vi "Kelvinox_Set_T_Setpoint.vi"(8 "error in (no error)":errorcluster, 10 "Kelvinox-Cluster":T2, 11 "Connection Details (in)":T1={"Mode"=enum."Immediate", "Bytes to Read"=5000, "IP Address"="172.25.187.107", "Remote Port"=33576, "Timeout"=10000, "connection ID"=refnum}) -> (0 "error out":errorcluster)   [LabVIEW 2019]
uses:
  Monitor Communication/Kelvinox/Kelvinox_Control.ctl
  Instrument_Setup.vi
panel:
  # "Pressures in mbar"
  # "Temperatures in K"
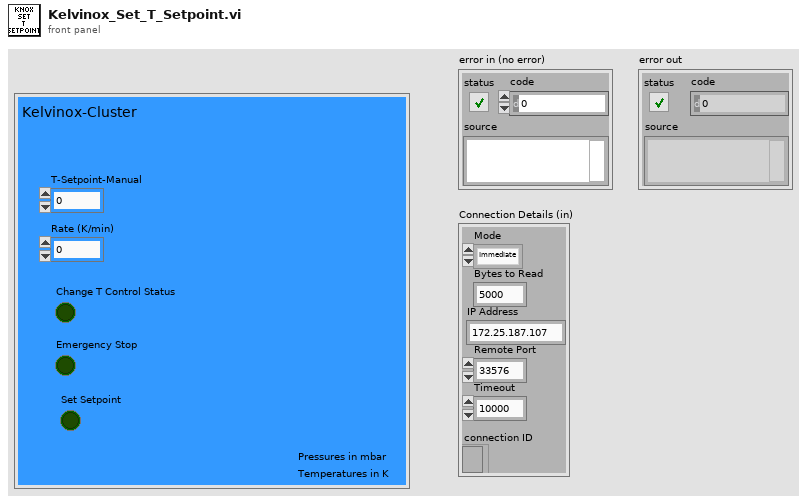
[diagram p1: front panel]
types:
  T1 = cluster{"Mode":enum16{"Standard", "Buffered", "CRLF", "Immediate"}, "Bytes to Read":i32, "IP Address":string, "Remote Port":i32, "Timeout":i32, "connection ID":refnum<k5>}
  T2 = typedef "Kelvinox_Control.ctl" = cluster{"T-Setpoint-Manual":dbl, "Rate (K/min)":dbl, "Change T Control Status":bool, "Emergency Stop":bool, "Set Setpoint":bool}
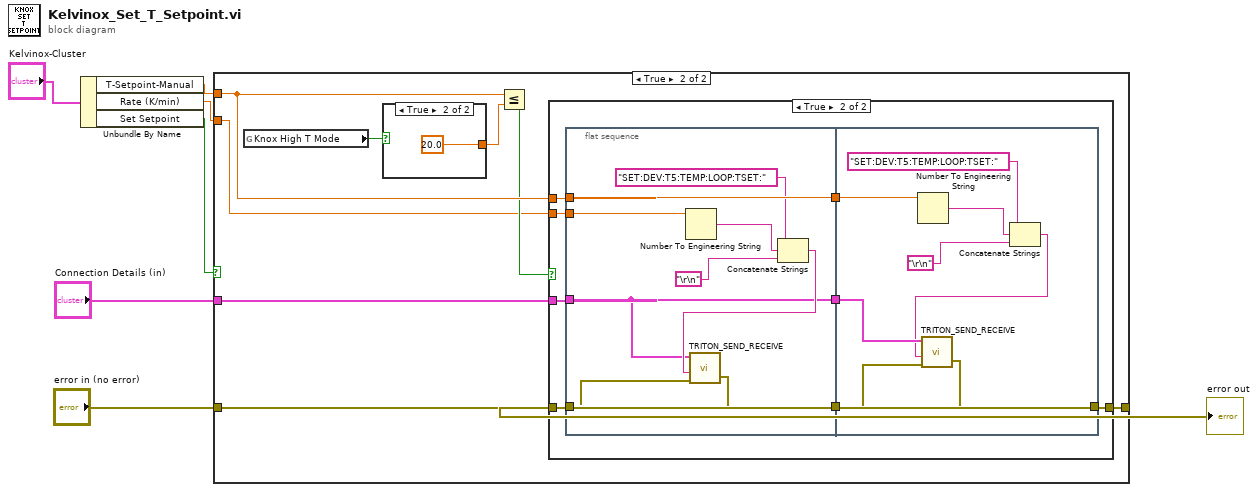
[diagram p0: block diagram]
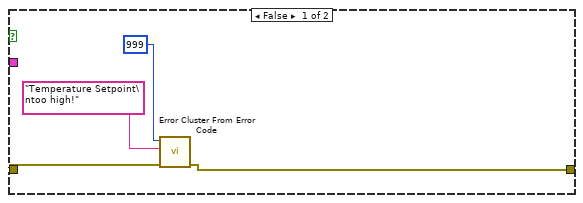
[diagram p3: hidden frame]
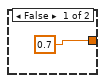
[diagram p4: hidden frame]
diagram:
  n1 = Unbundle By Name("Kelvinox-Cluster") -> ("T-Setpoint-Manual"=w2:dbl, "Rate (K/min)"=w1:dbl, "Set Setpoint"=w6:bool)
  n2 = case shown="True" w6 {
    tunnel: "error in (no error)" -> [w8 w16]
    tunnel: [w8 w15] -> w4
    tunnel: "Connection Details (in)" -> [_ w14]
    tunnel: w2 -> [_ w13]
    tunnel: w1 -> [_ w9]
    frame False {
    }
    frame True {
      n3 = global read "Instrument_Setup.vi" "Knox High T Mode"() -> (w12:bool)
      n4 = case shown="True" w12 {
        tunnel: [0.7 20.0] -> w11
        frame False {
        }
        frame True {
        }
      }
      n5 = Less Or Equal?(x=w13, y=w11) -> (x <= y?=w10:bool)
      n6 = case shown="True" w10 {
        tunnel: w16 -> [w18 w28]
        tunnel: [w17 w27] -> w15
        tunnel: w14 -> [_ w26]
        tunnel: w13 -> [_ w25]
        tunnel: w9 -> [_ w21]
        frame False {
          n7 = call <vilib>:"Error Cluster From Error Code.vi"("error in (no error)"=w18, "error message (\"\")"="Temperature Setpoint\ntoo high!", "error code (0)"=999) -> ("error out"=w17:errorcluster)  [unwired: 6 in]
        }
        frame True {
          n8 = flat-sequence {
            tunnel: w25 -> [w37]
            tunnel: w26 -> [w31]
            tunnel: w28 -> [w30]
            tunnel: [w29] -> w24
            tunnel: [w31] -> w23
            tunnel: [w37] -> w22
            tunnel: w21 -> [w32]
            tunnel: [w44] -> w27
            tunnel: w24 -> [w45]
            tunnel: w23 -> [w43]
            tunnel: w22 -> [w38]
            frame #0 {
              n9 = Number To Engineering String(4:w32) -> (0:w35:string)  [unwired: 3 in]
              n10 = Concatenate Strings("SET:DEV:T5:TEMP:LOOP:TSET:", w35, "\r\n") -> (w33:string)
              n11 = call "TRITON_SEND_RECEIVE.vi"("error in (no error)"=w30, "Command String"=w33, "Communication Cluster"=w31) -> ("error out"=w29:errorcluster)  [unwired: 1 in, 1 out]
            }
            frame #1 {
              n12 = Number To Engineering String(4:w38) -> (0:w41:string)  [unwired: 3 in]
              n13 = Concatenate Strings("SET:DEV:T5:TEMP:LOOP:TSET:", w41, "\r\n") -> (w39:string)
              n14 = call "TRITON_SEND_RECEIVE.vi"("error in (no error)"=w45, "Command String"=w39, "Communication Cluster"=w43) -> ("error out"=w44:errorcluster)  [unwired: 1 in, 1 out]
            }
          }
        }
      }
    }
  }
  "error out" <- w4
